vi "Pase String with TDs.vi"(8 "error in":errorcluster, 9 "Offset(0)":i32, 10 "Data String":string, 11 "Type Descriptors":cluster{T1}[](array[cluster])) -> (0 "error out":errorcluster, 1 "Offset Past Parsing":i32, 3 "Array of VData":variant[](array[variant]))   [LabVIEW 2012, in "TD Tools.lvlib"]
uses:
  TD Tools.lvlib
  Custom Type/Type Descriptor.ctl
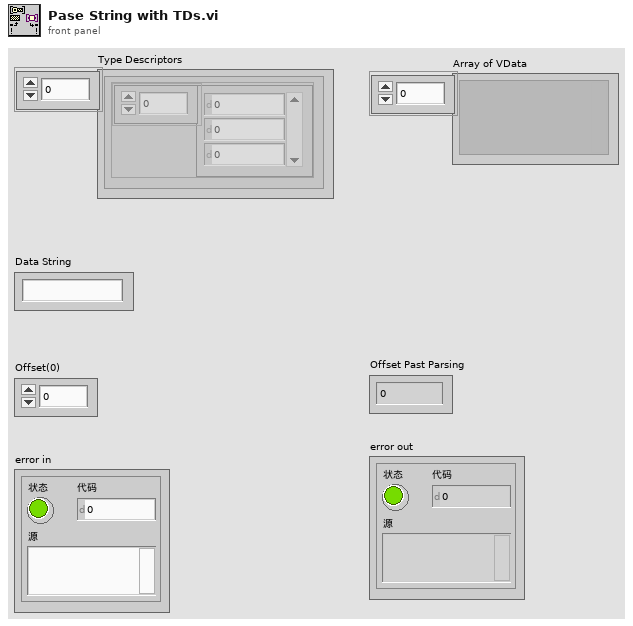
[diagram p1: front panel]
types:
  T1 = typedef "TD Tools.lvlib/Type Descriptor.ctl" = u16[]
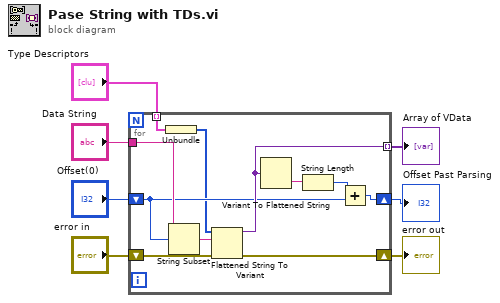
[diagram p0: block diagram]
diagram:
  n1 = for {
    tunnel: "Data String" -> [w15]
    tunnel: [w18] -> w5 mode=indexing
    shift-right: [w12] -> w3
    shift-left: "Offset(0)" -> [w14]
    shift-right: [w10] -> w1
    shift-left: "error in" -> [w11]
    tunnel: "Type Descriptors" -> [w9] mode=indexing
    n2 = Unbundle(w9) -> (w8:T1)
    n3 = String Subset(string=w15, offset (0)=w14) -> (substring=w16:string)  [unwired: 1 in]
    n4 = Flattened String To Variant(4:w11, 6:w16, 7:w8) -> (0:w10:errorcluster, 3:w18:variant)
    n5 = Variant To Flattened String(Variant=w18) -> (data string=w17:string)  [unwired: 1 out]
    n6 = String Length(string=w17) -> (length=w13:i32)
    n7 = Add(x=w13, y=w14) -> (x+y=w12:i32)
  }
  "Array of VData" <- w5
  "Offset Past Parsing" <- w3
  "error out" <- w1
